vi "Get New Tweets - Finite.vi"() -> ()   [LabVIEW 2011]
doc: "This example gets a finte number of new tweets starting from the top of the user's timeline.This example behaves the same way as Get Old Tweets- Finte if the Twitter Handle is not saved to a shift register."
uses:
  Controls/Tweet.ctl
  i3-twitter.lvlib
panel:
  out "Tweets":T1[](array[typedef])
  out "Time Stamp of Newest Tweet":timestamp
  in  "Screen Name (Empty)":string
  out "Num of Tweets Read":i32
  in  "Num of Tweets to Read (10)":i32=10
  in  "Consumer Key":string
  in  "Consumer Secret":string
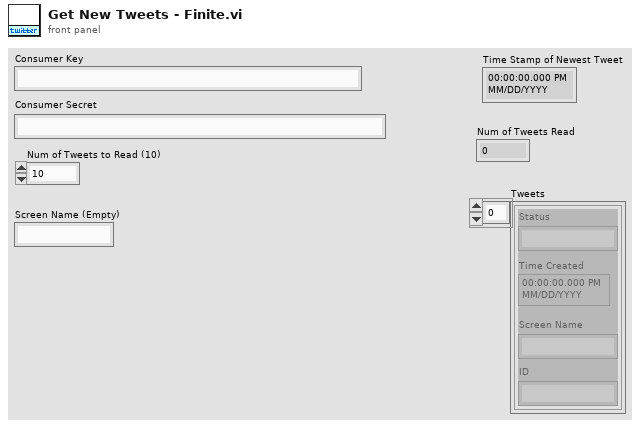
[diagram p1: front panel]
types:
  T1 = typedef "i3-twitter.lvlib/Tweet.ctl" = cluster{"Status":string, "Time Created":timestamp, "Screen Name":string, "ID":string}
  T2 = typedef "i3-oauth.lvlib/Credentials.ctl" = cluster{"Token":string, "Secret":string}
  T3 = typedef "i3-twitter.lvlib/Twitter Handle.ctl" = cluster{"OAuth Credentials":T4, "since ID":string, "max ID":string, "Screen Name":string}
  T4 = typedef "i3-oauth.lvlib/OAuth Handle.ctl" = cluster{"Signature Method":T5, "Version":string, "Client":T2, "Access":T2}
  T5 = typedef "i3-oauth.lvlib/Signature Method.ctl" = enum16{"HMAC-MD5", "HMAC-SHA1", "HMAC-SHA224", "HMAC-SHA256", "HMAC-SHA384", "HMAC-SHA512"}
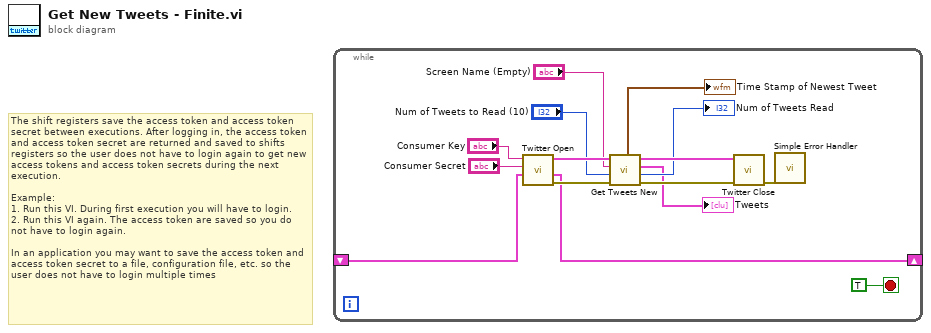
[diagram p0: block diagram]
diagram:
  # "The shift registers save the access token and access token secret between executions. After logging in, the access token and access token secret are returned and saved to shifts registers so the user does not have to login again to get new access tokens and access token secrets during the next execution.\n\nExample:\n1. Run this VI. During first execution you will have to login.\n2. Run this VI again. The access token are saved so you do not have to login again.\n\nIn an application you may want to save the access token and access token secret to a file, configuration file, etc. so the user does not have to login multiple times"
  n1 = while {
    shift-right: [w4] -> _
    shift-left: _ -> [w1]
    stop <- TRUE stop-if-true
    n2 = call "Twitter Open.vi"("Access Credentials (in)"=w1, "Consumer Secret"="Consumer Secret", "Consumer Key"="Consumer Key") -> ("error out"=w10:errorcluster, "Access Credentials (out)"=w4:T2, "Twitter Handle Out"=w13:T3)  [unwired: 6 in]
    n3 = call "Get Tweets New.vi"("error in"=w10, "Tweets to Read (10)"="Num of Tweets to Read (10)", "Screen Name (Empty)"="Screen Name (Empty)", "Twitter Handle In"=w13) -> ("error out"=w12:errorcluster, "Actual Num of Tweets Read"=→"Num of Tweets Read":i32, "New Tweets Read"=→"Tweets":T1[], "Twitter Handle Out"=w11:T3, "Time Stamp of Newest Tweet"=→"Time Stamp of Newest Tweet":timestamp)  [unwired: 3 in]
    n4 = call "Twitter Close.vi"("error in"=w12, "Twitter Handle In"=w11) -> ("error in"=w6:errorcluster)  [unwired: 9 in]
    n5 = call <vilib>:"Simple Error Handler.vi"("error in (no error)"=w6) -> ()  [unwired: 4 in, 5 out]
  }
